vi "Write Boolean.vi"(8 "error in (no error)":errorcluster, 10 "Boolean":bool=TRUE, 11 "Section 1 in":refnum<class "Section 1.lvclass">) -> (0 "error out":errorcluster, 3 "Section 1 out":refnum<class "Section 1.lvclass">)   [LabVIEW 2016, in "LVOOP Introduction.lvlib" / "Section 1.lvclass"]
uses:
  Section 1.lvclass
  Section 1.lvclass/Section 1.ctl
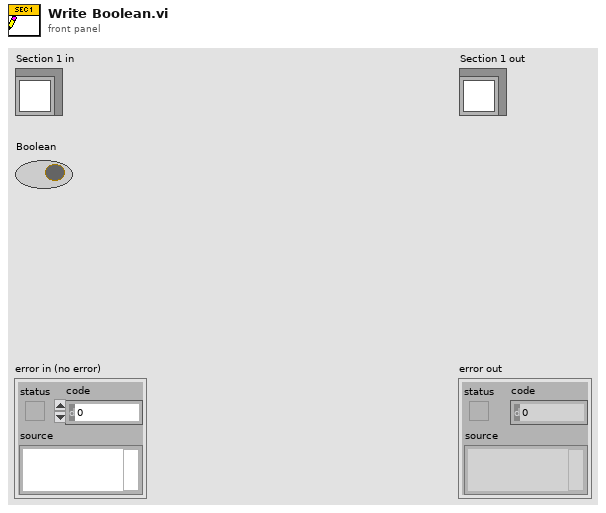
[diagram p1: front panel]
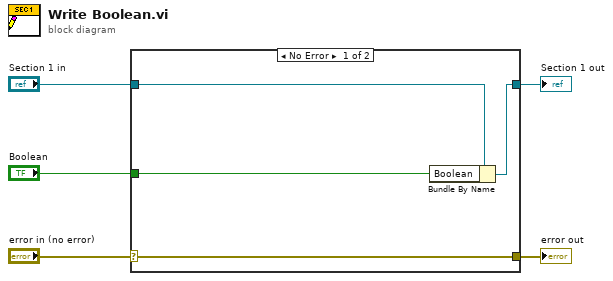
[diagram p0: block diagram]
diagram:
  n1 = case shown="No Error" "error in (no error)" {
    selector: "error in (no error)" -> [w9 w10]
    tunnel: [w9 w10] -> w4
    tunnel: [w7 w11] -> w2
    tunnel: "Section 1 in" -> [w8 w11]
    tunnel: "Boolean" -> [w6 _]
    frame No Error {
      n2 = Bundle By Name(cluster=w8, "Boolean"=w6) -> (w7:refnum<class "Section 1.lvclass">)
    }
    frame Error {
    }
  }
  "error out" <- w4
  "Section 1 out" <- w2
